vi "Abort Impl.vi"(8 "error in (no error)":errorcluster, 11 "ASI Stage in":refnum<class "ASI Stage.lvclass">) -> (0 "error out":errorcluster, 3 "ASI Stage out":refnum<class "ASI Stage.lvclass">)   [LabVIEW 2023, in "ASI Stage.lvlib" / "ASI Stage.lvclass"]
uses:
  ASI Stage.lvclass
  ASI Stage.lvclass/ASI Stage.ctl
  <instrlib>/ASI TG-1000/ASI TG-1000.lvlib
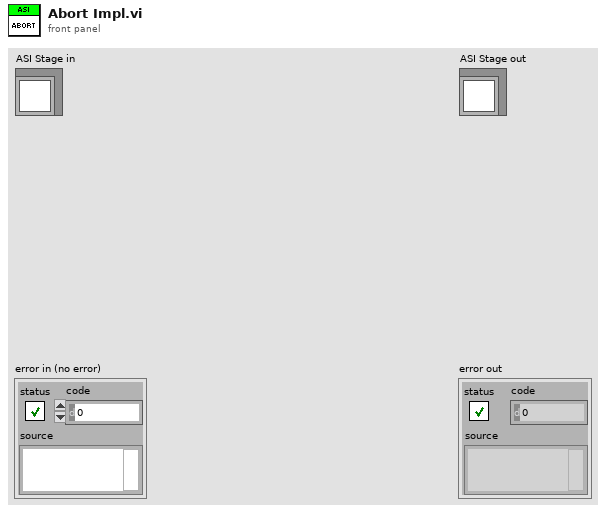
[diagram p1: front panel]
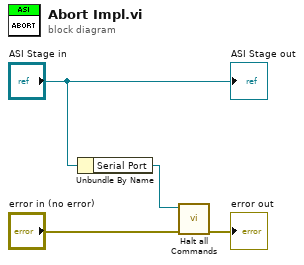
[diagram p0: block diagram]
diagram:
  n1 = Unbundle By Name("ASI Stage in") -> ("Serial Port"=w2:refnum<visa-resource-name>)
  n2 = call <instrlib>:"Halt all Commands.vi"("error in (no error)"="error in (no error)", "VISA in"=w2) -> ("error out"=→"error out":errorcluster)  [unwired: 7 in, 1 out]
  "ASI Stage out" <- "ASI Stage in"
